vi "CSM-FileSyncWindow.vi"(5 "Name(FileSync)":string="FileSync", 8 "error in":errorcluster) -> (0 "error out":errorcluster)   [LabVIEW 2020, in "CSM-FileSync.lvlib"]
doc: "------------- lvcsm -------------\n[CSMStates]\nItem 0 = \"Event Structure\"\nItem 1 = \"Idle\"\nItem 2 = \"CSM Documentation\"\nItem 3 = \"VI Reference\"\nItem 4 = \"Error Handler\"\nItem 5 = \"Critical Error\"\nItem 6 = \"Target Timeout Error\"\nItem 7 = \"Target Error\"\nItem 8 = \"Async Response\"\nItem 9 = \"Response\"\nItem 10 = \"Async Message Posted\"\nItem 11 = \"Initialize Core Data\"\nItem 12 = \"Exit\"\nItem 13 = \"Data: Initialize\"\nItem 14 = \"Data: Cleanup\"\nItem 15 = \"Events: Register\"\nItem 16 = \"Events: Unregister\"\nItem 17 = \"UI: Initialize\"\nItem 18 = \"UI: Cursor Set\"\nItem 19 = \"UI: Front Panel State\"\nItem 20 = \"Macro: Initialize\"\nItem 21 = \"Macro: Exit\"\nItem 22 = \"API: Update List\"\nItem 23 = \"API: Update Connected Status\"\nItem 24 = \"API: Update Statusbar\"\n\n[CSMStatus]\nItem 0 = \"Error Occurred@Error Handler\""
uses:
  CSM-FileSync.lvlib
  6641ad17-a0ad-4bac-bb5f-2ef3ab68202a.vi
  8cb7b144-fc6f-4ba1-ba8b-99306a1222b8.vi
  <userlib>/_NEVSTOP/Communicable State Machine(CSM)/AdvanceAPI/CSM - Revert Arguments-Safe String.vi
  <userlib>/_NEVSTOP/Communicable State Machine(CSM)/AdvanceAPI/CSM - Make String Arguments Safe.vi
  <userlib>/_NEVSTOP/Communicable State Machine(CSM)/AdvanceAPI/CSM - Break Down Multiple States String.vi
  <userlib>/_NEVSTOP/Communicable State Machine(CSM)/AdvanceAPI/CSM - Compact Multiple States.vi
  <userlib>/_NEVSTOP/Communicable State Machine(CSM)/AdvanceAPI/CSM - Keywords.vi
  <userlib>/_NEVSTOP/Communicable State Machine(CSM)/_Shared/Trim Single-line Text.vi
  <userlib>/_NEVSTOP/Communicable State Machine(CSM)/addons/MassData-Parameter/_support/FGV-MassData(lvlibp).vi
  <userlib>/_NEVSTOP/Communicable State Machine(CSM)/addons/API-String-Arugments-Support/_Support/Convert API String Arguments to Data(variant).vi
  <userlib>/_NEVSTOP/Communicable State Machine(CSM)/_Polymophic/CSM - Replace Marks in Messages.vi
  <userlib>/_NEVSTOP/Communicable State Machine(CSM)/Communicable State Machine.lvlib
  fb79005b-40a1-4b02-92b0-90b422e2c596.vi
panel:
  in  "Status":i32[](listbox)
  out "Statusbar":string
  out "Connected":bool
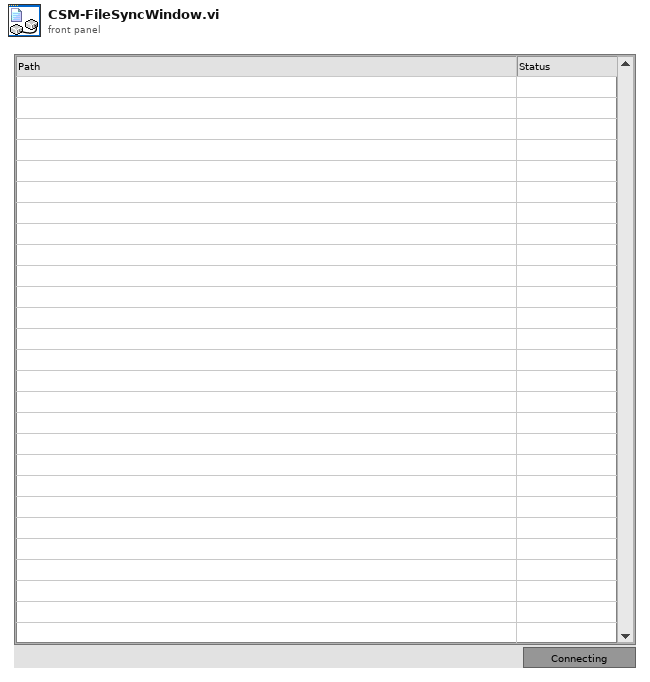
[diagram p1: front panel]
types:
  T1 = enum32{"Invalid", "Standard", "Closed", "Hidden", "Minimized", "Maximized"}
  T2 = enum32{"invalid app kind", "Development System", "Run Time System", "Student Edition", "Embedded LabVIEW", "Evaluation", "Custom"}
  T3 = cluster{"Upload List":path[], "UploadingFile":path}
  T4 = typedef "Communicable State Machine.lvlib/_CSM_Response Source Message.ctl" = cluster{"‘State":string, "’Arguments":string, "’Error":errorcluster}
  T5 = cluster{"Current VI Reference":refnum<vi>, "Close Panel on Exit?":bool}
  T6 = cluster{"Core":cluster{"Current VI Reference":refnum<vi>, "Close Panel on Exit?":bool}, "Status":refnum<vi>}
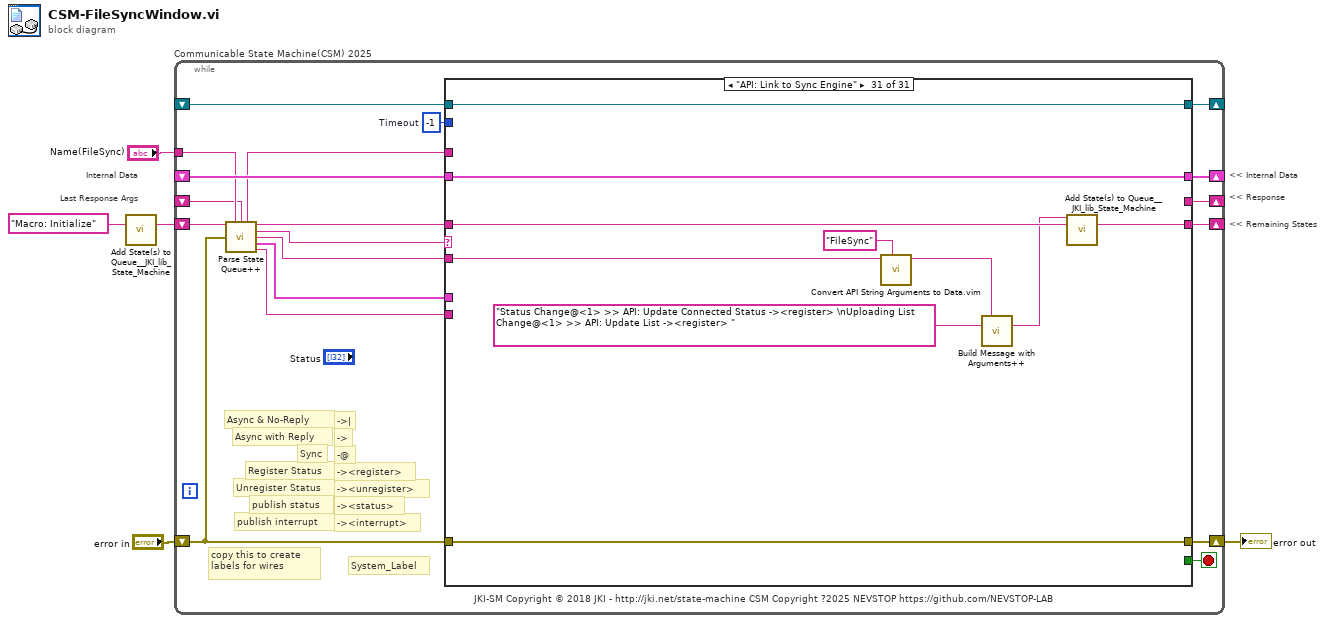
[diagram p0: block diagram]
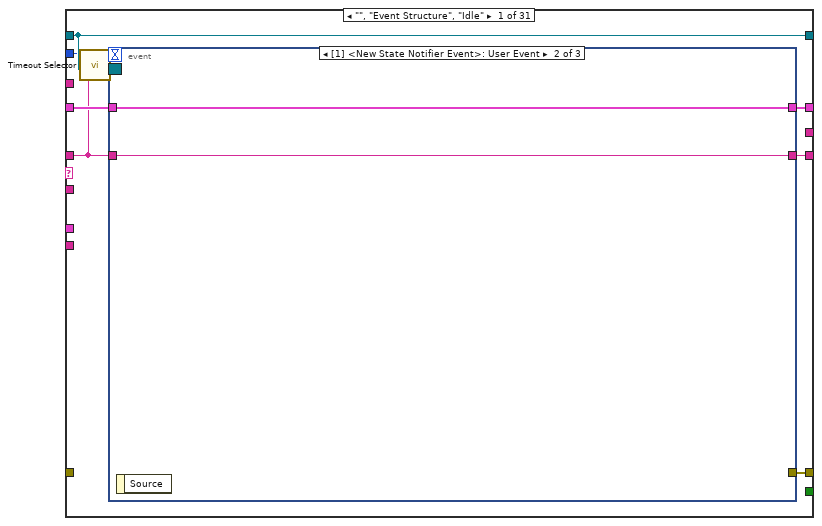
[diagram p2: hidden frame]
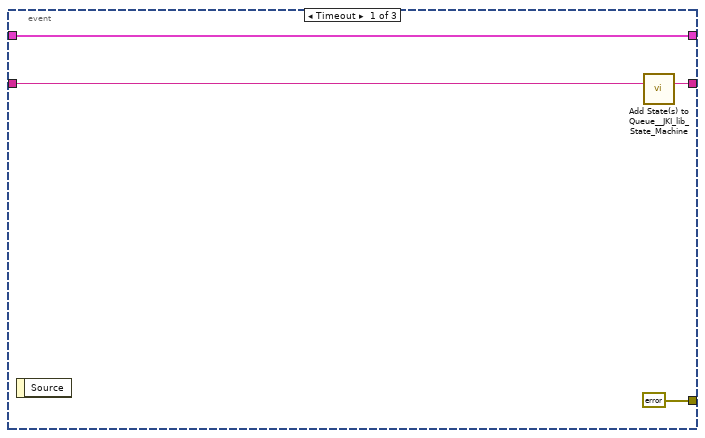
[diagram p3: hidden frame]
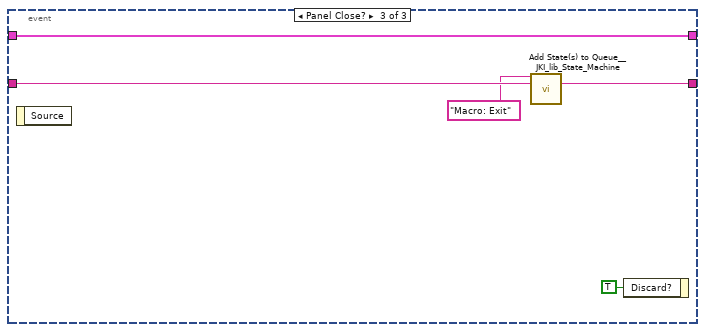
[diagram p4: hidden frame]
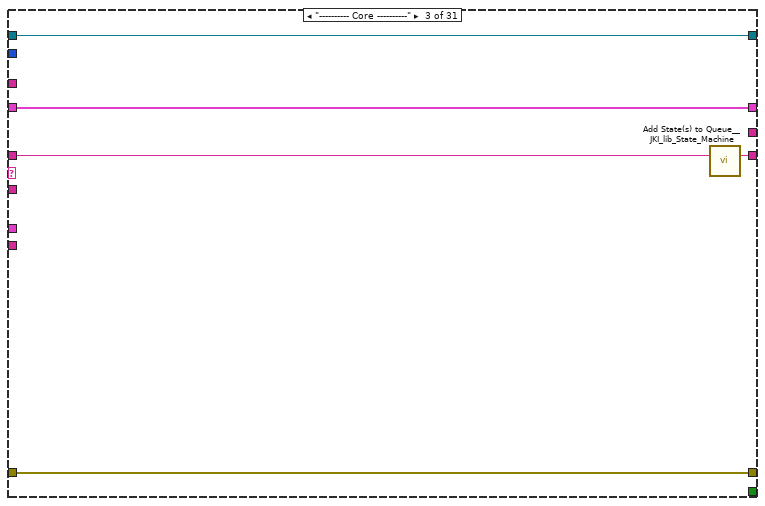
[diagram p6: hidden frame]
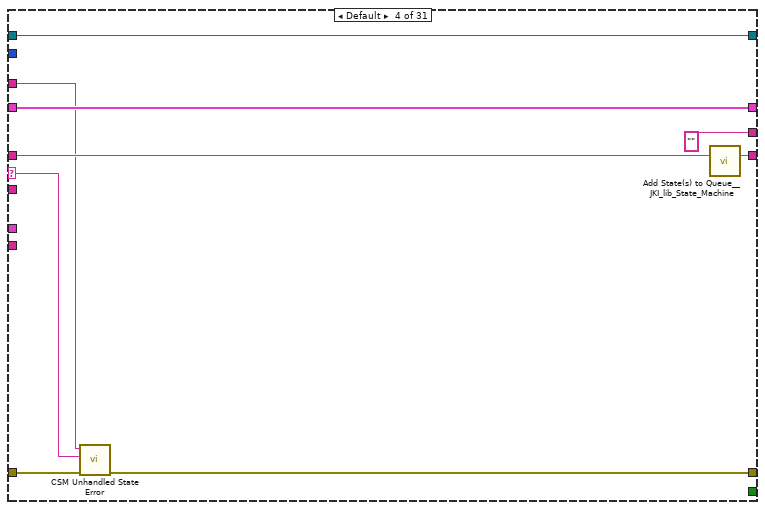
[diagram p7: hidden frame]
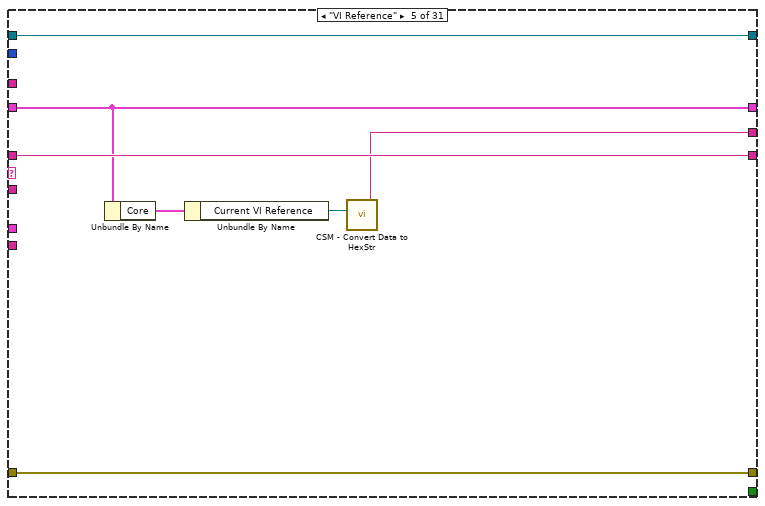
[diagram p8: hidden frame]
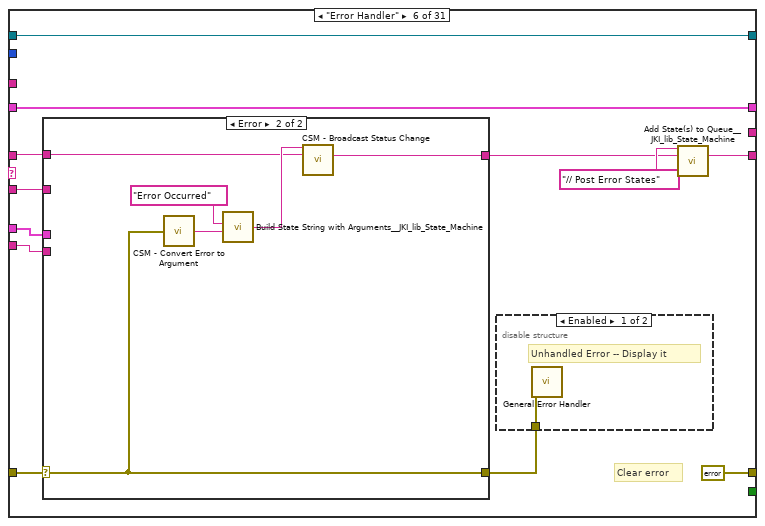
[diagram p9: hidden frame]
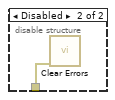
[diagram p10: hidden frame]
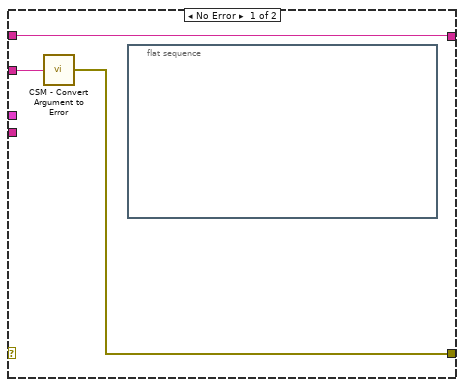
[diagram p11: hidden frame]
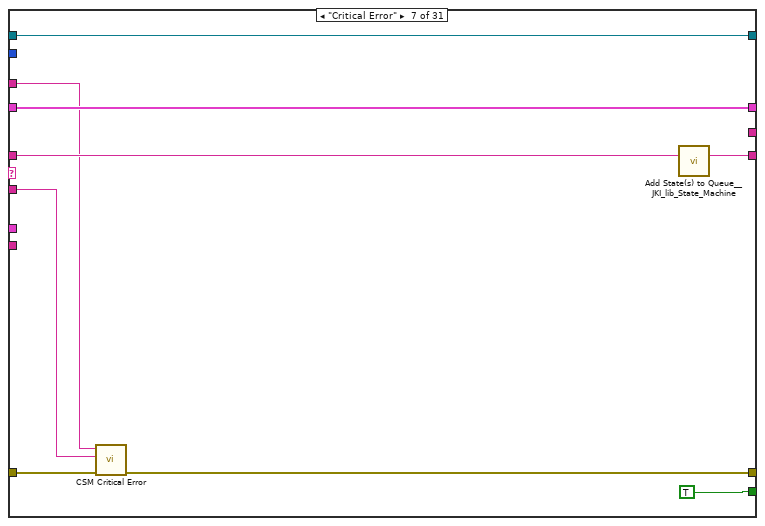
[diagram p12: hidden frame]
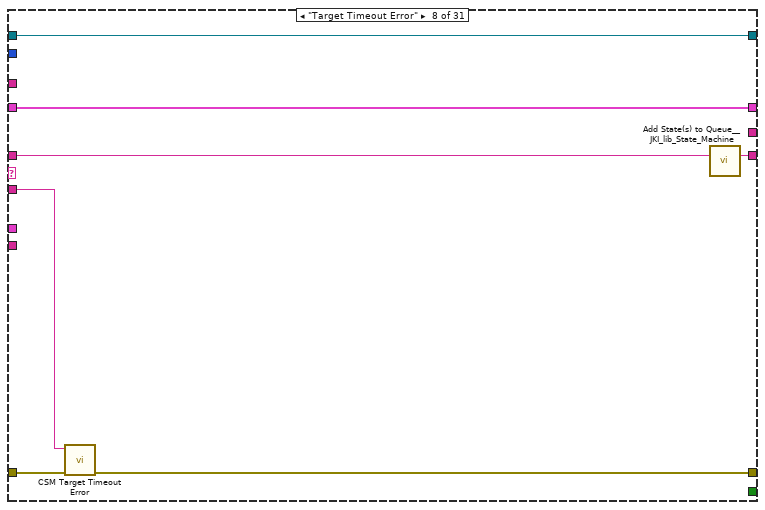
[diagram p13: hidden frame]
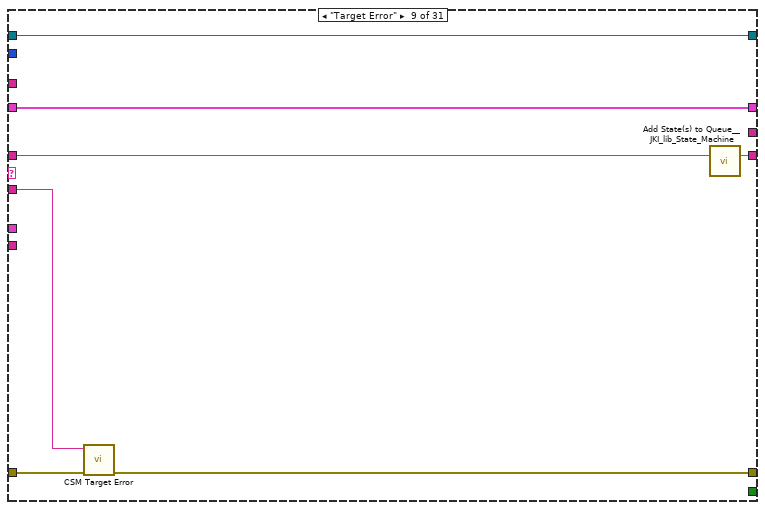
[diagram p14: hidden frame]
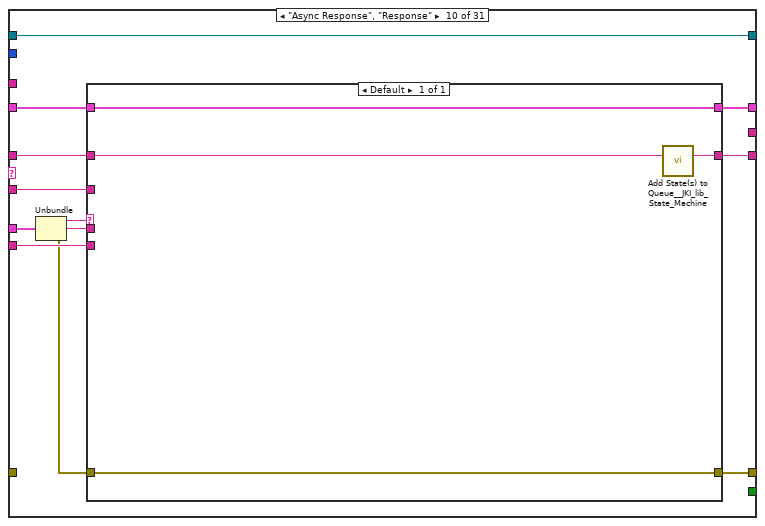
[diagram p15: hidden frame]
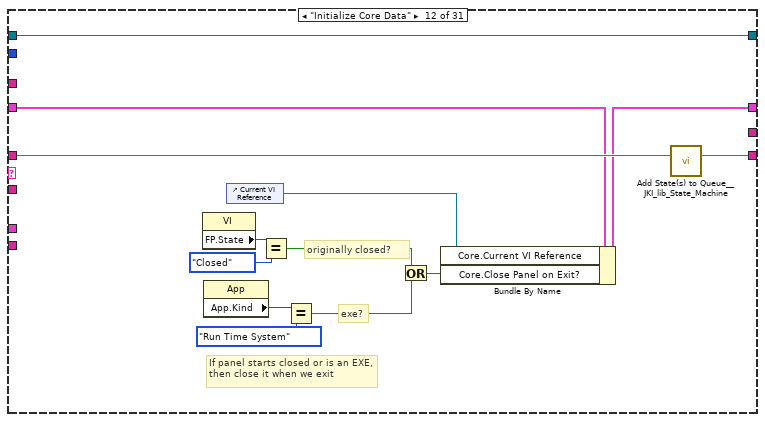
[diagram p17: hidden frame]
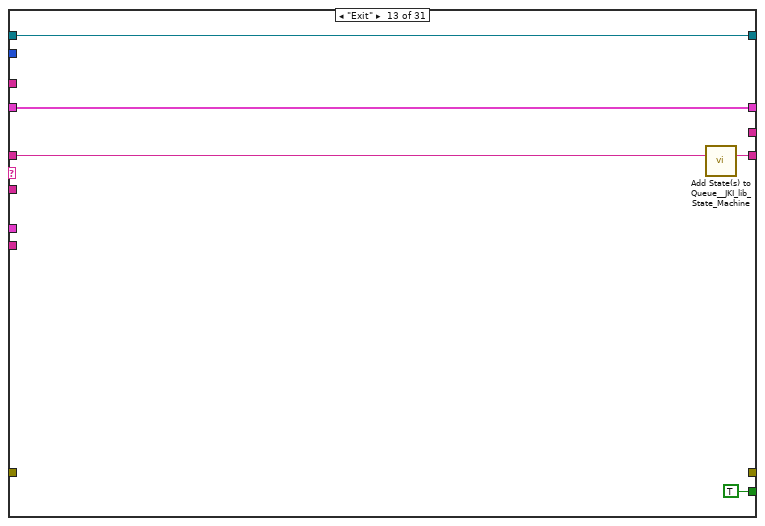
[diagram p18: hidden frame]
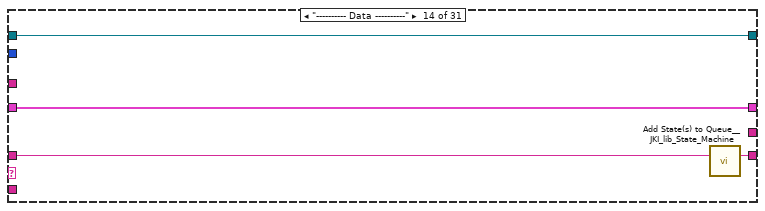
[diagram p19: hidden frame]
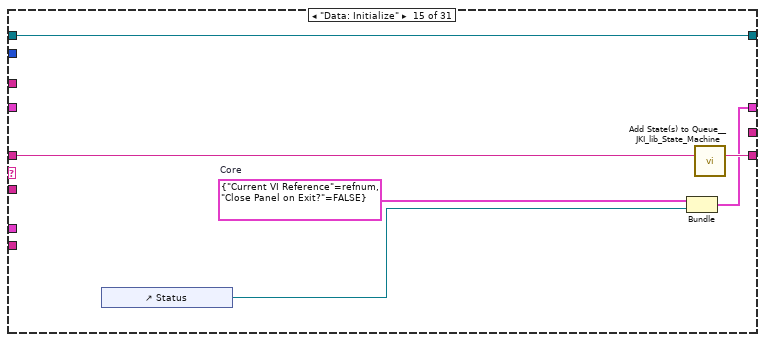
[diagram p20: hidden frame]
diagram:
  # "Last Response Args"
  # "Internal Data"
  # "<< Internal Data"
  # "<< Response"
  # "<< Remaining States"
  n1 = call <vilib>:"Add State(s) to Queue__JKI_lib_State_Machine.vi"("State(s) in (\"\")"="Macro: Initialize" ("Init State(\"Macro: Initialize\")")) -> ("States Out"=w4:string)  [unwired: 14 in]
  n2 = while "Communicable State Machine(CSM) 2025" {
    shift-right: [w19] -> _
    shift-left: _ -> [w18]
    shift-right: [w22] -> w1
    shift-left: "error in" -> [w16]
    shift-right: [w21] -> _
    shift-left: w4 -> [w23]
    tunnel: "Name(FileSync)" -> [w12]
    shift-right: [w15] -> _
    shift-left: _ -> [w7]
    shift-right: [w14] -> _
    shift-left: _ -> [w13]
    stop <- w20 stop-if-true
    w17 = -1  # Timeout
    # "-><interrupt>"
    # "-><status>"
    # "-><unregister>"
    # "-><register>"
    # "-@"
    # "->"
    # "->|"
    # "publish interrupt"
    # "publish status"
    # "Unregister Status"
    # "Register Status"
    # "Sync"
    # "Async with Reply"
    # "Async & No-Reply"
    # "copy this to create labels for wires"
    # "System_Label"
    # "JKI-SM Copyright © 2018 JKI - http://jki.net/state-machine CSM Copyright ?2025 NEVSTOP https://github.com/NEVSTOP-LAB"
    n3 = call <userlib>:"Parse State Queue++.vi"("State Queue"=w23, "Name (\"\" to Use UUID)"=w12, "Response Arguments"=w7, "Previous Error"=w16) -> ("Name Used"=w8:string, "Remaining States"=w24:string, "Current State"=w11:string, "Arguments"=w6:string, "Additional Information"=w10:T4, "Source CSM"=w9:string)  [unwired: 6 in]
    n4 = case shown="\"API: Link to Sync Engine\"" w11 {
      selector: w11 -> [_ _ _ w54 _ _ _ _ _ _ _ _ _ _ _ _ _ _ _ _ _ _ _ _ _ _ _ _ _ _ _]
      tunnel: w24 -> [w25 w46 w51 w60 w66 w72 w98 w106 w113 w123 w132 w145 w150 w154 w160 w166 w170 w177 w181 w185 w189 w195 w206 w270 w275 w286 w289 w301 w312 w317 w324]
      tunnel: w6 -> [_ _ _ _ _ w70 w94 w101 w109 w117 _ _ _ _ _ _ _ _ _ _ _ w191 w201 _ _ _ _ w299 w307 w314 w321]
      tunnel: w18 -> [w31 w45 w48 w58 w65 w78 w99 w104 w111 w121 w131 w139 w148 w152 _ w162 w168 w176 w180 w183 w187 w193 w203 w268 w273 w284 w288 w298 w311 w316 w327]
      tunnel: [w30 _ w49 w52 w67 errorcluster {"status"=FALSE, "code"=0, "source"=""} ("error out") w91 w100 w107 w120 _ _ _ _ _ w163 _ w171 w179 _ _ w192 w204 _ _ _ _ w297 w313 w318 w328] -> w22
      tunnel: w16 -> [_ _ w49 w53 w67 w76 w92 w102 w108 _ _ _ _ _ _ _ _ _ _ _ _ _ _ _ _ _ _ _ w313 w318 w328]
      tunnel: [w32 w46 w50 w59 w66 w74 w97 w105 w112 w124 w132 w144 w149 w153 w159 w165 w169 w177 w181 w184 w188 w194 w205 w269 w274 w285 w289 w301 w312 w317 w325] -> w21
      tunnel: [_ _ _ _ _ _ TRUE _ _ _ _ _ TRUE _ _ _ _ _ _ _ _ _ _ _ _ _ _ _ _ _ _] -> w20
      tunnel: [w29 w45 w48 w58 w65 w78 w99 w104 w111 w122 w131 w143 w148 w152 w158 w162 w168 w176 w180 w183 w187 w193 w203 w268 w273 w284 w288 w298 w311 w316 w327] -> w19
      tunnel: w17 -> [w27 _ _ _ _ _ _ _ _ _ _ _ _ _ _ _ _ _ _ _ _ _ _ _ _ _ _ _ _ _ _]
      tunnel: w9 -> [_ _ _ _ _ w69 _ _ _ w118 _ _ _ _ _ _ _ _ _ _ _ _ _ _ _ _ _ _ _ _ _]
      tunnel: w10 -> [_ _ _ _ _ w68 _ _ _ w119 _ _ _ _ _ _ _ _ _ _ _ _ _ _ _ _ _ _ _ _ _]
      tunnel: [_ _ _ "" w61 _ _ _ _ _ _ _ _ _ _ _ _ _ _ _ _ _ _ _ _ _ _ _ _ _ _] -> w15
      tunnel: [w28 w44 w47 w56 w64 w77 w95 w103 w110 w125 w130 w133 w146 w151 w156 w161 w167 w175 w178 w182 w186 w190 w200 w267 w271 w277 w287 w300 w310 w315 w326] -> w14
      tunnel: w13 -> [w28 w44 w47 w56 w64 w77 w95 w103 w110 w125 w130 w133 w146 w151 w156 w161 w167 _ w178 w182 w186 w190 w200 w267 w271 w277 w287 w300 w310 w315 w326]
      tunnel: w8 -> [_ _ _ w55 _ _ w93 _ _ _ _ _ _ _ _ _ _ w174 _ _ _ _ _ _ _ _ _ _ _ _ _]
      frame "", "Event Structure", "Idle" {
        n5 = call <userlib>:"Timeout Selector.vi"("Remaining States"=w25, "Timeout Expected"=w27) -> ("Timeout"=w26:i32)  [unwired: 5 in]
        n6 = event shown="[1] <New State Notifier Event>: User Event" {
          selector: w28 -> [_ _ _]
          dyn-events: _ -> [_ _ _]
          timeout: w26 -> [_ _ _]
          tunnel: w25 -> [w36 w37 w43]
          tunnel: [w35 w37 w42] -> w32
          tunnel: w31 -> [w34 w38 w41]
          tunnel: [errorcluster {"status"=FALSE, "code"=0, "source"=""} ("error out") _ _] -> w30
          tunnel: [w34 w38 w41] -> w29
          event Timeout {
            n7 = event-data() -> ()  [unwired: 1 in, 1 out]
            n8 = call <vilib>:"Add State(s) to Queue__JKI_lib_State_Machine.vi"("State(s) in (\"\")"=w36) -> ("States Out"=w35:string)  [unwired: 14 in]
          }
          event User Event {
            n9 = event-data() -> ()  [unwired: 1 in, 1 out]
          }
          event Panel Close? {
            n10 = event-data() -> ()  [unwired: 1 in, 1 out]
            n11 = call <vilib>:"Add State(s) to Queue__JKI_lib_State_Machine.vi"("State(s) in Front (\"\")"="Macro: Exit", "State(s) in (\"\")"=w43) -> ("States Out"=w42:string)  [unwired: 13 in]
            n12 = event-data("Discard?"=TRUE) -> ()  [unwired: 1 in, 1 out]
          }
        }
      }
      frame "CSM Documentation" {
      }
      frame "---------- Core ----------" {
        n13 = call <vilib>:"Add State(s) to Queue__JKI_lib_State_Machine.vi"("State(s) in (\"\")"=w51) -> ("States Out"=w50:string)  [unwired: 14 in]
      }
      frame Default {
        n14 = call <userlib>:"CSM Unhandled State Error.vi"("error in (no error)"=w53, "Undefined State"=w54, "CSM Name"=w55) -> ("error out"=w52:errorcluster)  [unwired: 8 in]
        n15 = call <vilib>:"Add State(s) to Queue__JKI_lib_State_Machine.vi"("State(s) in (\"\")"=w60) -> ("States Out"=w59:string)  [unwired: 14 in]
      }
      frame "VI Reference" {
        n16 = Unbundle By Name(w65) -> ("Core"=w63:T5)
        n17 = Unbundle By Name(w63) -> ("Current VI Reference"=w62:refnum<vi>)
        n18 = call <userlib>:"CSM - Convert Data to HexStr.vi"("Variant"=w62) -> ("HEX String (0-9,A-F)"=w61:string)  [unwired: 8 in]
      }
      frame "Error Handler" {
        # "Clear error"
        n19 = case shown="Error" w76 {
          selector: w76 -> [_ w85]
          tunnel: [w83 w87] -> w73
          tunnel: w72 -> [w83 w86]
          tunnel: [w82 w85] -> w71
          tunnel: w70 -> [w84 _]
          tunnel: w69 -> [_ _]
          tunnel: w68 -> [_ _]
          frame No Error {
            n20 = call <userlib>:"CSM - Convert Argument to Error.vi"("Argument"=w84) -> ("Error"=w82:errorcluster)  [unwired: 4 in]
            n21 = flat-sequence {
              frame #0 {
              }
            }
          }
          frame Error {
            n22 = call <userlib>:"CSM - Convert Error to Argument.vi"("Error"=w85) -> ("Argument"=w89:string)  [unwired: 4 in]
            n23 = call <vilib>:"Build State String with Arguments__JKI_lib_State_Machine.vi"("Arguments (\"\")"=w89, "State"="Error Occurred" ("Status with Arguments")) -> ("State with Arguments"=w88:string)  [unwired: 4 in]
            n24 = call <userlib>:"CSM - Broadcast Status Change.vi"("Status With Arguments"=w88, "State Queue"=w86) -> ("Remaining States"=w87:string)  [unwired: 13 in]
          }
        }
        n25 = disable-structure shown="Enabled" {
          disable-tunnel: w71 -> [w80 w81]
          frame Enabled {
            # "Unhandled Error -- Display it"
            n26 = call <vilib>:"General Error Handler.vi"("error in (no error)"=w80) -> ()  [unwired: 10 in, 5 out]
          }
          frame Disabled {
            n27 = call <vilib>:"Clear Errors.vi"("error in (no error)"=w81) -> ()  [unwired: 5 in, 2 out]
          }
        }
        n28 = call <vilib>:"Add State(s) to Queue__JKI_lib_State_Machine.vi"("State(s) in Front (\"\")"="// Post Error States", "State(s) in (\"\")"=w73) -> ("States Out"=w74:string)  [unwired: 13 in]
      }
      frame "Critical Error" {
        n29 = call <userlib>:"CSM Critical Error.vi"("error in (no error)"=w92, "Arugments (As Reason)"=w94, "CSM Name"=w93) -> ("error out"=w91:errorcluster)  [unwired: 8 in]
        n30 = call <vilib>:"Add State(s) to Queue__JKI_lib_State_Machine.vi"("State(s) in (\"\")"=w98) -> ("States Out"=w97:string)  [unwired: 14 in]
      }
      frame "Target Timeout Error" {
        n31 = call <userlib>:"CSM Target Timeout Error.vi"("error in (no error)"=w102, "Arguments (As CSM Name)"=w101) -> ("error out"=w100:errorcluster)  [unwired: 9 in]
        n32 = call <vilib>:"Add State(s) to Queue__JKI_lib_State_Machine.vi"("State(s) in (\"\")"=w106) -> ("States Out"=w105:string)  [unwired: 14 in]
      }
      frame "Target Error" {
        n33 = call <userlib>:"CSM Target Error.vi"("error in (no error)"=w108, "Arguments (As CSM Name)"=w109) -> ("error out"=w107:errorcluster)  [unwired: 9 in]
        n34 = call <vilib>:"Add State(s) to Queue__JKI_lib_State_Machine.vi"("State(s) in (\"\")"=w113) -> ("States Out"=w112:string)  [unwired: 14 in]
      }
      frame "Async Response", "Response" {
        n35 = Unbundle(w119) -> ("‘State"=w116:string, "’Arguments"=w115:string, "’Error"=w114:errorcluster)
        n36 = case shown="Default" w116 {
          tunnel: [w126] -> w124
          tunnel: w123 -> [w127]
          tunnel: [w129] -> w122
          tunnel: w121 -> [w129]
          tunnel: [w128] -> w120
          tunnel: w114 -> [w128]
          tunnel: w118 -> [_]
          tunnel: w117 -> [_]
          tunnel: w115 -> [_]
          frame Default {
            n37 = call <vilib>:"Add State(s) to Queue__JKI_lib_State_Machine.vi"("State(s) in (\"\")"=w127) -> ("States Out"=w126:string)  [unwired: 14 in]
          }
        }
      }
      frame "Async Message Posted" {
      }
      frame "Initialize Core Data" {
        # "originally closed?"
        # "exe?"
        # "If panel starts closed or is an EXE, then close it when we exit"
        n38 = property class="VI"() -> ("FP.State"=w136:T1)  [unwired: 2 in, 2 out]
        n39 = property class="App"() -> ("App.Kind"=w142:T2)  [unwired: 2 in, 2 out]
        n40 = control-ref of="Current VI Reference"() -> (w137:refnum<vi>)
        n41 = Equal?(x=w136, y=T1."Closed" ("Front Panel Window:State")) -> (x = y?=w134:bool)
        n42 = Equal?(x=w142, y=T2."Run Time System" ("Application:Kind")) -> (x = y?=w140:bool)
        n43 = Or(x=w134, y=w140) -> (x .or. y?=w138:bool)
        n44 = Bundle By Name(cluster=w139, "Core.Current VI Reference"=w137, "Core.Close Panel on Exit?"=w138) -> (w143:T6)
        n45 = call <vilib>:"Add State(s) to Queue__JKI_lib_State_Machine.vi"("State(s) in (\"\")"=w145) -> ("States Out"=w144:string)  [unwired: 14 in]
      }
      frame "Exit" {
        n46 = call <vilib>:"Add State(s) to Queue__JKI_lib_State_Machine.vi"("State(s) in (\"\")"=w150) -> ("States Out"=w149:string)  [unwired: 14 in]
      }
      frame "---------- Data ----------" {
        n47 = call <vilib>:"Add State(s) to Queue__JKI_lib_State_Machine.vi"("State(s) in (\"\")"=w154) -> ("States Out"=w153:string)  [unwired: 14 in]
      }
      frame "Data: Initialize" {
        w157 = T5 {"Current VI Reference"=refnum, "Close Panel on Exit?"=FALSE}  # Core
        n48 = control-ref of="Status"() -> (w155:refnum<vi>)
        n49 = Bundle("Core"=w157, "Status"=w155) -> (w158:T6)  [unwired: 1 in]
        n50 = call <vilib>:"Add State(s) to Queue__JKI_lib_State_Machine.vi"("State(s) in (\"\")"=w160) -> ("States Out"=w159:string)  [unwired: 14 in]
      }
      frame "Data: Cleanup" {
        n51 = Unbundle By Name(w162) -> ("Core.Current VI Reference"=w164:refnum<vi>)
        n52 = Close Reference(reference=w164) -> (error out=w163:errorcluster)  [unwired: 1 in]
        n53 = call <vilib>:"Add State(s) to Queue__JKI_lib_State_Machine.vi"("State(s) in (\"\")"=w166) -> ("States Out"=w165:string)  [unwired: 14 in]
      }
      frame "---------- Events ----------" {
        n54 = call <vilib>:"Add State(s) to Queue__JKI_lib_State_Machine.vi"("State(s) in (\"\")"=w170) -> ("States Out"=w169:string)  [unwired: 14 in]
      }
      frame "Events: Register" {
        n55 = call <userlib>:"CSM - Get New State Notifier Event.vi"("Name (\"\" to Use UUID)"=w174) -> ("error out"=w172:errorcluster, "New State Notifier Event"=w173:refnum<user-event>)  [unwired: 9 in]
        n56 = register-events(error in=w172, w173) -> (reference out=w175:refnum<event-registration>, error out=w171:errorcluster)  [unwired: 1 in]
      }
      frame "Events: Unregister" {
        n57 = Unregister For Events(event registration refnum=w178) -> (error out=w179:errorcluster)  [unwired: 1 in]
      }
      frame "---------- UI ----------" {
        n58 = call <vilib>:"Add State(s) to Queue__JKI_lib_State_Machine.vi"("State(s) in (\"\")"=w185) -> ("States Out"=w184:string)  [unwired: 14 in]
      }
      frame "UI: Initialize" {
        n59 = call <vilib>:"Add State(s) to Queue__JKI_lib_State_Machine.vi"("State(s) in (\"\")"=w189) -> ("States Out"=w188:string)  [unwired: 14 in]
      }
      frame "UI: Cursor Set" {
        # "Argument"
        n60 = disable-structure shown="TARGET_TYPE!=Windows" {
          disable-tunnel: [w197 _] -> w192
          disable-tunnel: w191 -> [w196 _]
          frame condition #0 (active) {
            n61 = case shown="\"Idle\", Default" w196 {
              tunnel: [w198 w199] -> w197
              frame "Idle", Default {
                n62 = call <vilib>:"Unset Busy.vi"() -> ("error out"=w198:errorcluster)  [unwired: 11 in]
              }
              frame "Busy" {
                n63 = call <vilib>:"Set Busy.vi"() -> ("error out"=w199:errorcluster)  [unwired: 10 in, 1 out]
              }
            }
          }
          frame condition #1 {
          }
        }
        n64 = call <vilib>:"Add State(s) to Queue__JKI_lib_State_Machine.vi"("State(s) in (\"\")"=w195) -> ("States Out"=w194:string)  [unwired: 14 in]
      }
      frame "UI: Front Panel State" {
        # "Argument"
        n65 = Unbundle By Name(w203) -> ("Core.Current VI Reference"=w202:refnum<vi>)
        n66 = case shown="\"Minimize\", \"Minimized\"" w201 {
          tunnel: [w213 w226 w237 w249 w261] -> w204
          tunnel: w202 -> [w212 w224 w236 w248 w260]
          frame "Open", "Standard", Default {
            w207 = T1."Standard" ("State")
            n67 = property class="VI"(reference=w212) -> (reference out=w210:refnum<vi>, error out=w211:errorcluster, "FP.State"=w209:T1)  [unwired: 1 in]
            n68 = Not Equal?(x=w209, y=w207) -> (x != y?=w208:bool)
            n69 = case shown="True" w208 {
              tunnel: [w217 w219] -> w213
              tunnel: w211 -> [w216 w219]
              tunnel: w210 -> [w215 _]
              tunnel: w207 -> [w214 _]
              frame True {
                n70 = invoke class="VI" method="FP.Open"(reference=w215, error in=w216, "Activate"=TRUE, "State"=w214) -> (error out=w217:errorcluster)  [unwired: 1 in, 4 out]
              }
              frame False {
              }
            }
          }
          frame "Close", "Closed" {
            n71 = property class="VI"(reference=w224) -> (reference out=w223:refnum<vi>, error out=w225:errorcluster, "FP.State"=w221:T1)  [unwired: 1 in]
            n72 = Not Equal?(x=w221, y=T1."Closed" ("Front Panel Window:State")) -> (x != y?=w220:bool)
            n73 = case shown="True" w220 {
              tunnel: [w227 w230] -> w226
              tunnel: w225 -> [w227 w229]
              tunnel: w223 -> [_ w228]
              frame False {
              }
              frame True {
                n74 = invoke class="VI" method="FP.Close"(reference=w228, error in=w229) -> (error out=w230:errorcluster)  [unwired: 1 in, 2 out]
              }
            }
          }
          frame "Hidden", "Hide" {
            w231 = T1."Hidden" ("State")
            n75 = property class="VI"(reference=w236) -> (reference out=w234:refnum<vi>, error out=w235:errorcluster, "FP.State"=w233:T1)  [unwired: 1 in]
            n76 = Not Equal?(x=w233, y=w231) -> (x != y?=w232:bool)
            n77 = case shown="True" w232 {
              tunnel: [w241 w242] -> w237
              tunnel: w235 -> [w240 w242]
              tunnel: w234 -> [w239 _]
              tunnel: w231 -> [w238 _]
              frame True {
                n78 = invoke class="VI" method="FP.Open"(reference=w239, error in=w240, "State"=w238) -> (error out=w241:errorcluster)  [unwired: 2 in, 4 out]
              }
              frame False {
              }
            }
          }
          frame "Minimize", "Minimized" {
            w243 = T1."Minimized" ("State")
            n79 = property class="VI"(reference=w248) -> (reference out=w246:refnum<vi>, error out=w247:errorcluster, "FP.State"=w245:T1)  [unwired: 1 in]
            n80 = Not Equal?(x=w245, y=w243) -> (x != y?=w244:bool)
            n81 = case shown="False" w244 {
              tunnel: [w253 w254] -> w249
              tunnel: w247 -> [w252 w254]
              tunnel: w246 -> [w251 _]
              tunnel: w243 -> [w250 _]
              frame True {
                n82 = invoke class="VI" method="FP.Open"(reference=w251, error in=w252, "State"=w250) -> (error out=w253:errorcluster)  [unwired: 2 in, 4 out]
              }
              frame False {
              }
            }
          }
          frame "Maximize", "Maximized" {
            w255 = T1."Maximized" ("State")
            n83 = property class="VI"(reference=w260) -> (reference out=w258:refnum<vi>, error out=w259:errorcluster, "FP.State"=w257:T1)  [unwired: 1 in]
            n84 = Not Equal?(x=w257, y=w255) -> (x != y?=w256:bool)
            n85 = case shown="True" w256 {
              tunnel: [w265 w266] -> w261
              tunnel: w259 -> [w264 w266]
              tunnel: w258 -> [w263 _]
              tunnel: w255 -> [w262 _]
              frame True {
                n86 = invoke class="VI" method="FP.Open"(reference=w263, error in=w264, "State"=w262) -> (error out=w265:errorcluster)  [unwired: 2 in, 4 out]
              }
              frame False {
              }
            }
          }
        }
        n87 = call <vilib>:"Add State(s) to Queue__JKI_lib_State_Machine.vi"("State(s) in (\"\")"=w206) -> ("States Out"=w205:string)  [unwired: 14 in]
      }
      frame "---------- Macro ----------" {
        n88 = call <vilib>:"Add State(s) to Queue__JKI_lib_State_Machine.vi"("State(s) in (\"\")"=w270) -> ("States Out"=w269:string)  [unwired: 14 in]
      }
      frame "Macro: Initialize" {
        w272 = "Data: Initialize\nInitialize Core Data\nEvents: Register\nUI: Initialize\nUI: Front Panel State >> Open"  # Data: Initialize Initialize Core Data Events: Register UI: Initialize UI: Front Panel State >> Open
        n89 = call <vilib>:"Add State(s) to Queue__JKI_lib_State_Machine.vi"("State(s) in Front (\"\")"=w272, "State(s) in (\"\")"=w275) -> ("States Out"=w274:string)  [unwired: 13 in]
      }
      frame "Macro: Exit" {
        n90 = Unbundle By Name(w284) -> ("Core.Close Panel on Exit?"=w283:bool)
        n91 = Select(t="UI: Front Panel State >> Close", s=w283, f="") -> (s? t:f=w280:string)
        n92 = call <vilib>:"Add State(s) to Queue__JKI_lib_State_Machine.vi"("State(s) in Front (\"\")"="//Exit Sub-Modules ", "State(s) in (\"\")"=w280, "State(s) at Back (\"\")"="Data: Cleanup\nEvents: Unregister\nExit") -> ("States Out"=w278:string)  [unwired: 12 in]
        n93 = call <vilib>:"Add State(s) to Queue__JKI_lib_State_Machine.vi"("State(s) in Front (\"\")"=w278, "State(s) in (\"\")"=w286) -> ("States Out"=w285:string)  [unwired: 13 in]
      }
      frame "---------- API ----------" {
      }
      frame "API: Update List" {
        n94 = Unbundle By Name(w298) -> ("Status"=w295:refnum<vi>)
        n95 = call "CSM - Convert Argument to MassData.vim"("Type"=T3 {"Upload List"=[], "UploadingFile"=path ""} ("output cluster"), "MassData Argument"=w299) -> ("error out"=w297:errorcluster, "Data"=w294:T3)  [unwired: 6 in]
        n96 = feedback-in #1(w294) -> ()
        n97 = feedback #1() -> (w293:T3)  [unwired: 1 in]
        n98 = Not Equal?(x=w294, y=w293) -> (x != y?=w291:bool)
        n99 = First Call?() -> (First Call?: T/F=w290:bool)
        n100 = Or(x=w291, y=w290) -> (x .or. y?=w292:bool)
        n101 = case shown="True" w292 {
          tunnel: w295 -> [_ w304]
          tunnel: w294 -> [_ w303]
          frame False {
          }
          frame True {
            n102 = Unbundle(w303) -> ("Upload List"=w306:path[], "UploadingFile"=w305:path)
            n103 = call "Prepare Status Table.vi"("MulticolumnListbox in"=w304, "Temp:UploadingFile"=w305, "Upload List"=w306) -> ("Array"=w302:string[][])  [unwired: 8 in]
            n104 = property class="MCListbox (strict)"(reference=w304, "ItemNames"=w302) -> ()  [unwired: 1 in, 2 out]
          }
        }
      }
      frame "API: Update Connected Status" {
        n105 = call "Convert API String Arguments to Data.vim"("Reference Type"=FALSE, "API String"=w307) -> ("Data"=→"Connected":bool)  [unwired: 6 in, 1 out]
      }
      frame "API: Update Statusbar" {
        "Statusbar" <- w314
      }
      frame "API: Link to Sync Engine" {
        n106 = call "Convert API String Arguments to Data.vim"("Reference Type"="FileSync" ("Name(FileSync)"), "API String"=w321) -> ("Data"=w319:string)  [unwired: 6 in, 1 out]
        n107 = call-poly <userlib>:"Build Message with Arguments++.vi"("States With Replace Token"="Status Change@<1> >> API: Update Connected Status -><register> \nUploading List Change@<1> >> API: Update List -><register> " ("State(s) in Front (\"\")"), "<1>"=w319) -> ("States"=w322:string)  [unwired: 13 in]
        n108 = call <vilib>:"Add State(s) to Queue__JKI_lib_State_Machine.vi"("State(s) in Front (\"\")"=w322, "State(s) in (\"\")"=w324) -> ("States Out"=w325:string)  [unwired: 13 in]
      }
    }
  }
  "error out" <- w1
